vi "LVClass_WavefrontCorrectorSet get initial actuators specifications.vi"(0 "WavefrontCorrectorSet in":refnum<class "WavefrontCorrectorSet.lvclass">, 11 "error in (no error)":errorcluster) -> (4 "WavefrontCorrectorSet out":refnum<class "WavefrontCorrectorSet.lvclass">, 6 "Wavefront Corrector State":T1[](array[typedef]), 15 "error out":errorcluster)   [LabVIEW 2020, in "WavefrontCorrectorSet.lvclass"]
doc: "WavefrontCorrector constraints getter.\n\n--------------------------------------------------------------------------------\n\n<B>wavefrontcorrector_setIn </B> : WavefrontCorrectorSet object.\n<B>wavefrontcorrector_setOut </B> : WavefrontCorrectorSet object.\n<B>max </B> : WavefrontCorrector preferences : highest command value. See\n cWavefrontCorrector.\n<B>min </B> : WavefrontCorrector preferences : lowest command value. See\n cWavefrontCorrector.\n<B>validity </B> : WavefrontCorrector preferences : status. See cWavefrontCorrector.\n<B>position </B> : WavefrontCorrector preferences : fixed positions. See cWavefrontCorrector.\n<B>ErrorIn </B> : Error\n<B>ErrorOut </B> : Error\n\n--------------------------------------------------------------------------------"
uses:
  WavefrontCorrectorSet.lvclass
  Wavefront Corrector states - ONE.ctl
  WavefrontCorrectorSet.lvclass/WavefrontCorrectorSet.ctl
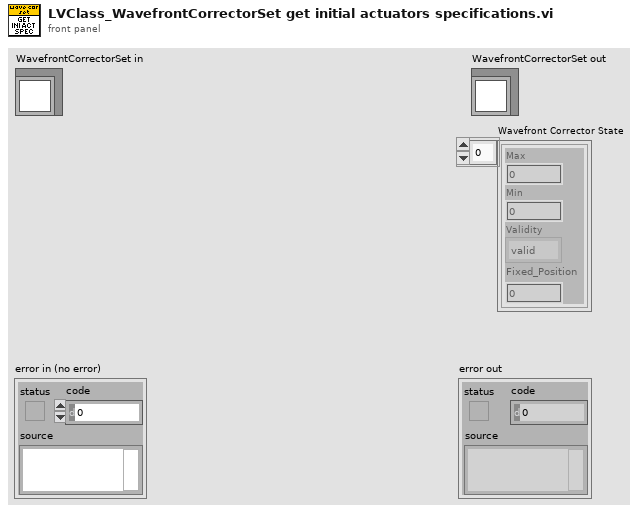
[diagram p1: front panel]
types:
  T1 = typedef "Wavefront Corrector states - ONE.ctl" = cluster{"Max":sgl, "Min":sgl, "Validity":enum16{"valid", "fixed", "invalid"}, "Fixed_Position":sgl}
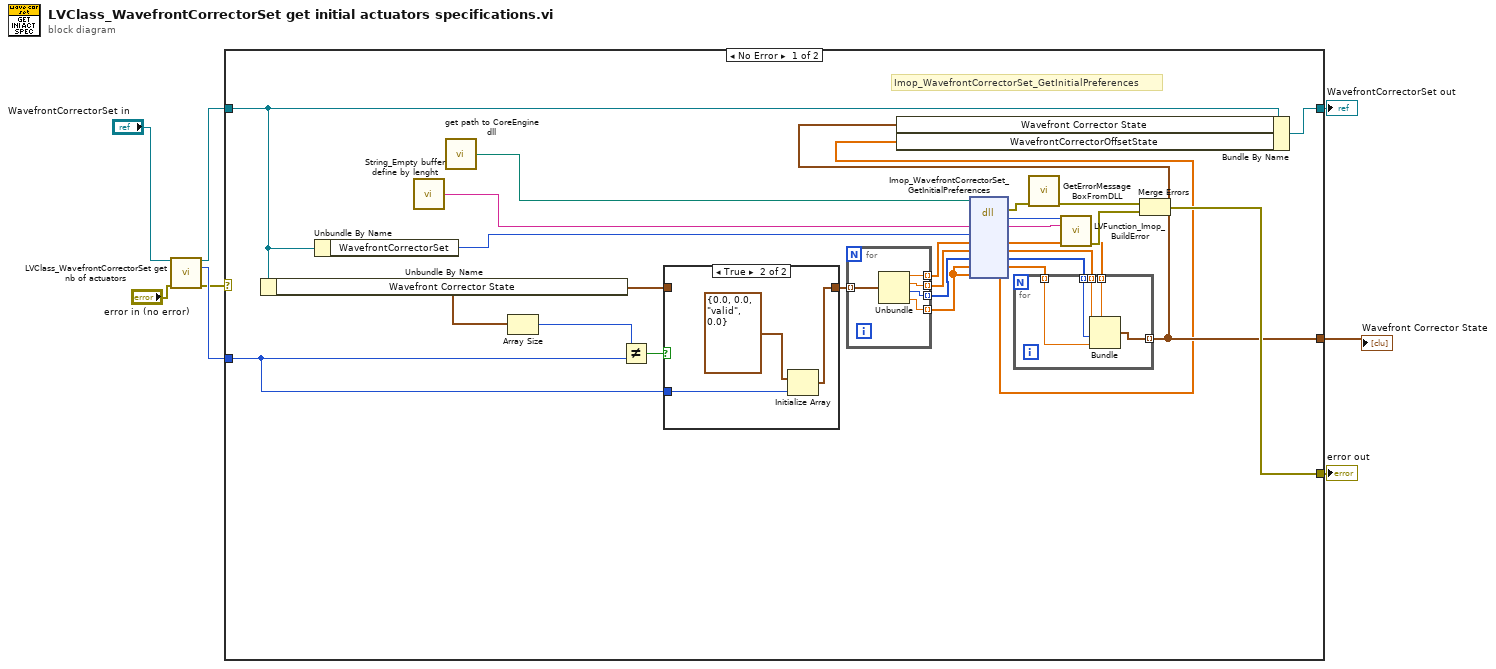
[diagram p0: block diagram]
diagram:
  n1 = call "LVClass_WavefrontCorrectorSet get nb of actuators.vi"("WavefrontCorrectorSet in"="WavefrontCorrectorSet in", "error in (no error)"="error in (no error)") -> ("WavefrontCorrectorSet out"=w2:refnum<class "WavefrontCorrectorSet.lvclass">, "ActuatorsNumber"=w6:i32, "error out"=w4:errorcluster)  [unwired: 11 in]
  n2 = case shown="No Error" w4 {
    selector: w4 -> [_ w50]
    tunnel: [w26 w50] -> w8
    tunnel: [w13 w49] -> w7
    tunnel: w2 -> [w14 w49]
    tunnel: w6 -> [w18 _]
    tunnel: [w11 _] -> w1
    frame No Error {
      # "Imop_WavefrontCorrectorSet_GetInitialPreferences"
      n3 = Unbundle By Name(w14) -> ("Wavefront Corrector State"=w19:T1[])
      n4 = Unbundle By Name(w14) -> ("WavefrontCorrectorSet"=w27:i32)
      n5 = call "String_Empty buffer define by lenght.vi"() -> ("Empty buffer"=w32:string)  [unwired: 1 in]
      n6 = call "get path to CoreEngine dll.vi"() -> ("path to c_interface_vc100.dll"=w31:path)  [unwired: 12 in, 3 out]
      n7 = Array Size(array=w19) -> (size(s)=w9:i32)
      n8 = Not Equal?(x=w9, y=w18) -> (x != y?=w21:bool)
      n9 = case shown="True" w21 {
        tunnel: [w40 w42] -> w20
        tunnel: w18 -> [_ w43]
        tunnel: w19 -> [w40 _]
        frame False {
        }
        frame True {
          n10 = Initialize Array(T1 {"Max"=0.0, "Min"=0.0, "Validity"=enum."valid", "Fixed_Position"=0.0} ("Actuator state"), w43) -> (w42:T1[])
        }
      }
      n11 = for {
        tunnel: w20 -> [w39] mode=indexing
        tunnel: [w38] -> w17 mode=indexing
        tunnel: [w37] -> w16 mode=indexing
        tunnel: [w36] -> w15 mode=indexing
        tunnel: [w35] -> w12 mode=indexing
        n12 = Unbundle(w39) -> ("Max"=w38:sgl, "Min"=w37:sgl, "Validity"=w36:enum16{"valid", "fixed", "invalid"}, "Fixed_Position"=w35:sgl)
      }
      n13 = dll-call lib="D:/soft/HASO_v3/C_interface/Sources/Build/vc100/Release/c_interface_vc100.dll" fn="Imop_WavefrontCorrectorSet_GetInitialPreferences"(path in=w31, "message"=w32, "WavefrontCorrectionSet"=w27, "Tab max"=w17, "tab min"=w16, "tab validity"=w15, "fixed_values"=w12, "init_positions"=w12) -> (error out=w30:errorcluster, "return type"=w34:i32, "message"=w33:string, "Tab max"=w25:sgl[], "tab min"=w24:sgl[], "tab validity"=w23:i32[], "fixed_values"=w22:sgl[], "init_positions"=w10:sgl[])  [unwired: 3 in, 1 out]
      n14 = for {
        tunnel: w25 -> [w48] mode=indexing
        tunnel: w24 -> [w47] mode=indexing
        tunnel: w23 -> [w46] mode=indexing
        tunnel: w22 -> [w45] mode=indexing
        tunnel: [w44] -> w11 mode=indexing
        n15 = Bundle(w48, w47, w46, w45) -> (w44:cluster{sgl, sgl, i32, sgl})  [unwired: 1 in]
      }
      n16 = Bundle By Name(cluster=w14, "Wavefront Corrector State"=w11, "WavefrontCorrectorOffsetState"=w10) -> (w13:refnum<class "WavefrontCorrectorSet.lvclass">)
      n17 = call "GetErrorMessageBoxFromDLL.vi"("error IN"=w30) -> ("error OUT"=w29:errorcluster)  [unwired: 10 in]
      n18 = call "LVFunction_Imop_BuildError.vi"("code"=w34, "String to Prepend to source (\"\")"=w33) -> ("error out"=w28:errorcluster)  [unwired: 13 in]
      n19 = Merge Errors(w29, w28) -> (w26:errorcluster)
    }
    frame Error {
    }
  }
  "error out" <- w8
  "WavefrontCorrectorSet out" <- w7
  "Wavefront Corrector State" <- w1
